vi "OFDM_SuperpositionedBitDetect_TDMA.vi"(0 "Input symbols":cdb[](array[numeric]) format="%.2f", 1 "Modulation type":T1(ring), 3 "error in (no error)":errorcluster) -> (5 "Base Bits":i8[](array[numeric]), 6 "SC Symbols":cdb[](array[numeric]), 7 "SC Bits":i8[](array[numeric]), 10 "error out":errorcluster)   [LabVIEW 2022 SP3]
uses:
  <vilib>/addons/Modulation/Digital/General/MT Map QAM Symbols to Bits.vi
  <vilib>/addons/Modulation/Digital/General/MT Map Bits to QAM Symbols.vi
  <vilib>/addons/Modulation/Digital/General/MT Map PSK Symbols to Bits.vi
  <vilib>/addons/Modulation/Digital/General/MT Map Bits to PSK Symbols.vi
  <vilib>/addons/Modulation/niDMT.lvlib
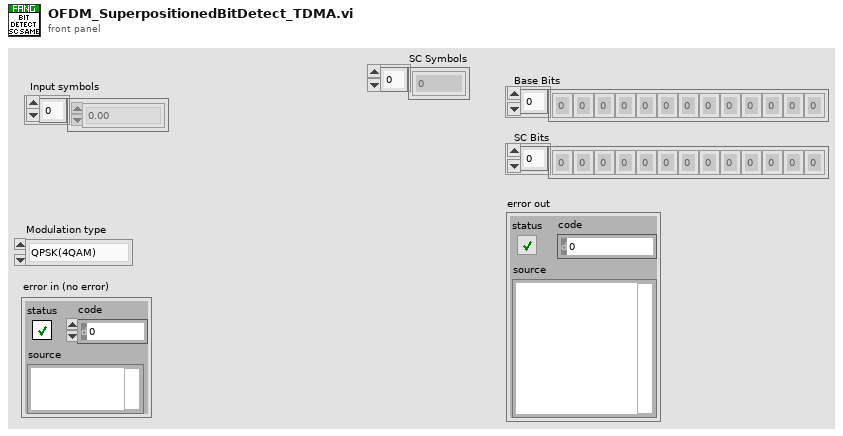
[diagram p1: front panel]
types:
  T1 = enum16{"QPSK(4QAM)", "64QAM", "16QAM", "BPSK", "BPSK Vertical"}
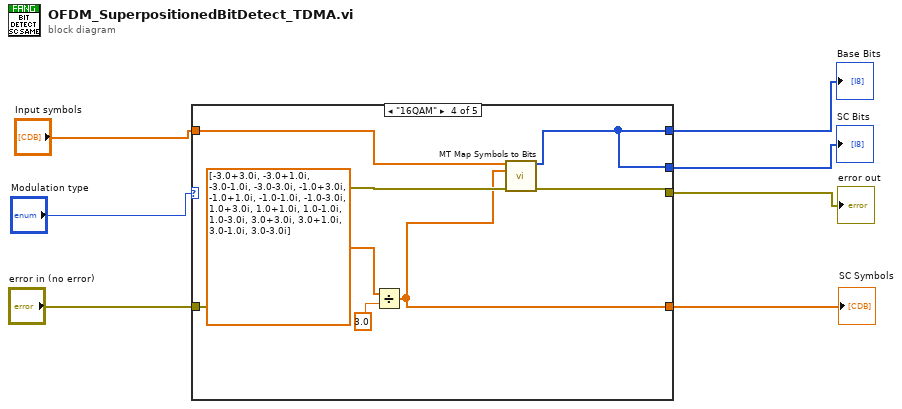
[diagram p0: block diagram]
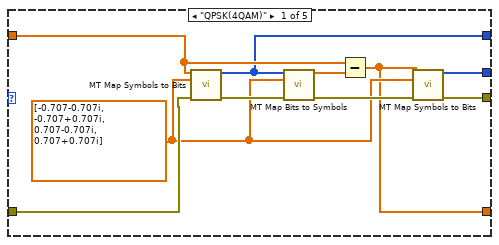
[diagram p2: hidden frame]
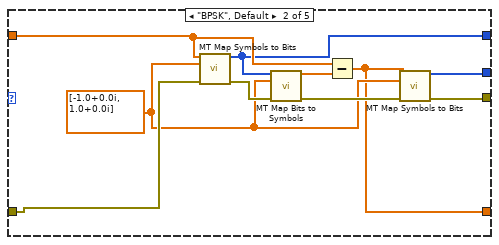
[diagram p3: hidden frame]
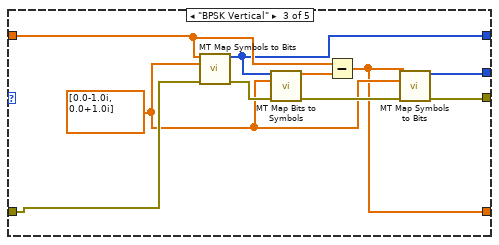
[diagram p4: hidden frame]
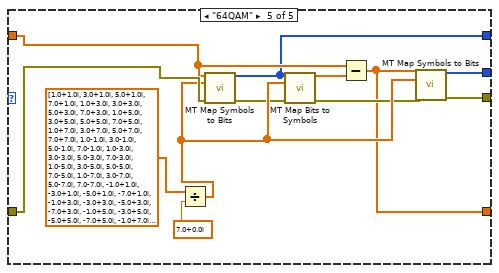
[diagram p5: hidden frame]
diagram:
  n1 = case shown="\"16QAM\"" "Modulation type" {
    tunnel: "Input symbols" -> [w14 w20 w30 w39 w51]
    tunnel: "error in (no error)" -> [w17 w27 w37 w44 w54]
    tunnel: [w10 w23 w33 w40 w50] -> w4
    tunnel: [w12 w24 w34 w41 w49] -> w3
    tunnel: [w9 w19 w29 w40 w46] -> w2
    tunnel: [w8 w18 w28 w38 w45] -> w1
    frame "QPSK(4QAM)" {
      w11 = cdb[] [-0.707-0.707i, -0.707+0.707i, 0.707-0.707i, 0.707+0.707i] ("symbol map")
      n2 = call-poly <vilib>:"MT Map Symbols to Bits.vi"("symbols"=w14, "symbol map"=w11, "error in (no error)"=w17) -> ("output bit stream"=w9:i8[], "error out"=w16:errorcluster)  [unwired: 11 in]
      n3 = call-poly <vilib>:"MT Map Bits to Symbols.vi"("input bit stream"=w9, "symbol map"=w11, "error in (no error)"=w16) -> ("symbols"=w15:cdb[], "error out"=w13:errorcluster)  [unwired: 11 in]
      n4 = Subtract(x=w14, y=w15) -> (x-y=w8:cdb[])
      n5 = call-poly <vilib>:"MT Map Symbols to Bits.vi"("symbols"=w8, "symbol map"=w11, "error in (no error)"=w13) -> ("output bit stream"=w10:i8[], "error out"=w12:errorcluster)  [unwired: 11 in]
    }
    frame "BPSK", Default {
      w22 = cdb[] [-1.0+0.0i, 1.0+0.0i] ("symbol map")
      n6 = call-poly <vilib>:"MT Map Symbols to Bits.vi"("symbols"=w20, "symbol map"=w22, "error in (no error)"=w27) -> ("output bit stream"=w19:i8[], "error out"=w26:errorcluster)  [unwired: 11 in]
      n7 = call-poly <vilib>:"MT Map Bits to Symbols.vi"("input bit stream"=w19, "symbol map"=w22, "error in (no error)"=w26) -> ("symbols"=w21:cdb[], "error out"=w25:errorcluster)  [unwired: 11 in]
      n8 = Subtract(x=w20, y=w21) -> (x-y=w18:cdb[])
      n9 = call-poly <vilib>:"MT Map Symbols to Bits.vi"("symbols"=w18, "symbol map"=w22, "error in (no error)"=w25) -> ("output bit stream"=w23:i8[], "error out"=w24:errorcluster)  [unwired: 11 in]
    }
    frame "BPSK Vertical" {
      w32 = cdb[] [0.0-1.0i, 0.0+1.0i] ("symbol map")
      n10 = call-poly <vilib>:"MT Map Symbols to Bits.vi"("symbols"=w30, "symbol map"=w32, "error in (no error)"=w37) -> ("output bit stream"=w29:i8[], "error out"=w36:errorcluster)  [unwired: 11 in]
      n11 = call-poly <vilib>:"MT Map Bits to Symbols.vi"("input bit stream"=w29, "symbol map"=w32, "error in (no error)"=w36) -> ("symbols"=w31:cdb[], "error out"=w35:errorcluster)  [unwired: 11 in]
      n12 = Subtract(x=w30, y=w31) -> (x-y=w28:cdb[])
      n13 = call-poly <vilib>:"MT Map Symbols to Bits.vi"("symbols"=w28, "symbol map"=w32, "error in (no error)"=w35) -> ("output bit stream"=w33:i8[], "error out"=w34:errorcluster)  [unwired: 11 in]
    }
    frame "16QAM" {
      n14 = Divide(x=cdb[] [-3.0+3.0i, -3.0+1.0i, -3.0-1.0i, -3.0-3.0i, -1.0+3.0i, -1.0+1.0i, -1.0-1.0i, -1.0-3.0i, 1.0+3.0i, 1.0+1.0i, 1.0-1.0i, 1.0-3.0i, 3.0+3.0i, 3.0+1.0i, 3.0-1.0i, 3.0-3.0i] ("symbol map"), y=3.0) -> (x/y=w38:cdb[])
      n15 = call-poly <vilib>:"MT Map Symbols to Bits.vi"("symbols"=w39, "symbol map"=w38, "error in (no error)"=w44) -> ("output bit stream"=w40:i8[], "error out"=w41:errorcluster)  [unwired: 11 in]
    }
    frame "64QAM" {
      n16 = Divide(x=cdb[] [1.0+1.0i, 3.0+1.0i, 5.0+1.0i, 7.0+1.0i, 1.0+3.0i, 3.0+3.0i, 5.0+3.0i, 7.0+3.0i, 1.0+5.0i, 3.0+5.0i, 5.0+5.0i, 7.0+5.0i, 1.0+7.0i, 3.0+7.0i, 5.0+7.0i, 7.0+7.0i, 1.0-1.0i, 3.0-1.0i, 5.0-1.0i, 7.0-1.0i, 1.0-3.0i, 3.0-3.0i, 5.0-3.0i, 7.0-3.0i, 1.0-5.0i, 3.0-5.0i, 5.0-5.0i, 7.0-5.0i, 1.0-7.0i, 3.0-7.0i, 5.0-7.0i, 7.0-7.0i, -1.0+1.0i, -3.0+1.0i, -5.0+1.0i, -7.0+1.0i, -1.0+3.0i, -3.0+3.0i, -5.0+3.0i, -7.0+3.0i, -1.0+5.0i, -3.0+5.0i, -5.0+5.0i, -7.0+5.0i, -1.0+7.0i, -3.0+7.0i, -5.0+7.0i, -7.0+7.0i, -1.0-1.0i, -3.0-1.0i, -5.0-1.0i, -7.0-1.0i, -1.0-3.0i, -3.0-3.0i, -5.0-3.0i, -7.0-3.0i, -1.0-5.0i, -3.0-5.0i, -5.0-5.0i, -7.0-5.0i, -1.0-7.0i, -3.0-7.0i, -5.0-7.0i, -7.0-7.0i] ("appended array"), y=cdb 7.0+0.0i) -> (x/y=w53:cdb[])
      n17 = call-poly <vilib>:"MT Map Symbols to Bits.vi"("symbols"=w51, "symbol map"=w53, "error in (no error)"=w54) -> ("output bit stream"=w46:i8[], "error out"=w48:errorcluster)  [unwired: 11 in]
      n18 = call-poly <vilib>:"MT Map Bits to Symbols.vi"("input bit stream"=w46, "symbol map"=w53, "error in (no error)"=w48) -> ("symbols"=w52:cdb[], "error out"=w47:errorcluster)  [unwired: 11 in]
      n19 = Subtract(x=w51, y=w52) -> (x-y=w45:cdb[])
      n20 = call-poly <vilib>:"MT Map Symbols to Bits.vi"("symbols"=w45, "symbol map"=w53, "error in (no error)"=w47) -> ("output bit stream"=w50:i8[], "error out"=w49:errorcluster)  [unwired: 11 in]
    }
  }
  "SC Bits" <- w4
  "error out" <- w3
  "Base Bits" <- w2
  "SC Symbols" <- w1
